vi "TEG P116x1_Write_Manual.vi"(8 "error in (no error)":errorcluster, 9 "NewRT":dbl, 10 "NewSP":dbl, 11 "Comunicaciones":T1={"EUROTHERM"="ASRL6::INSTR", "eur"=FALSE, "ESP32"="ASRL6::INSTR", "esp"=FALSE}) -> (0 "error out":errorcluster, 1 "NewRT 2":dbl, 2 "NewSP 2":dbl)   [LabVIEW 2017]
uses:
  cTEG COMMS.ctl
  Eurotherm_New_Module.ctl
  TEG TEST 2022 GLOBALES.vi
panel:
  out "PV":dbl
  out "WorKSP":dbl
  out "TargetSP":dbl
  in  "Cancel":bool
  in  "Write":bool
  out "Enable(T)":bool=TRUE
  out "VISA Promux":refnum<visa-resource-name>
  # "Programando controlador P116"
  # "C"
  # "C/min"
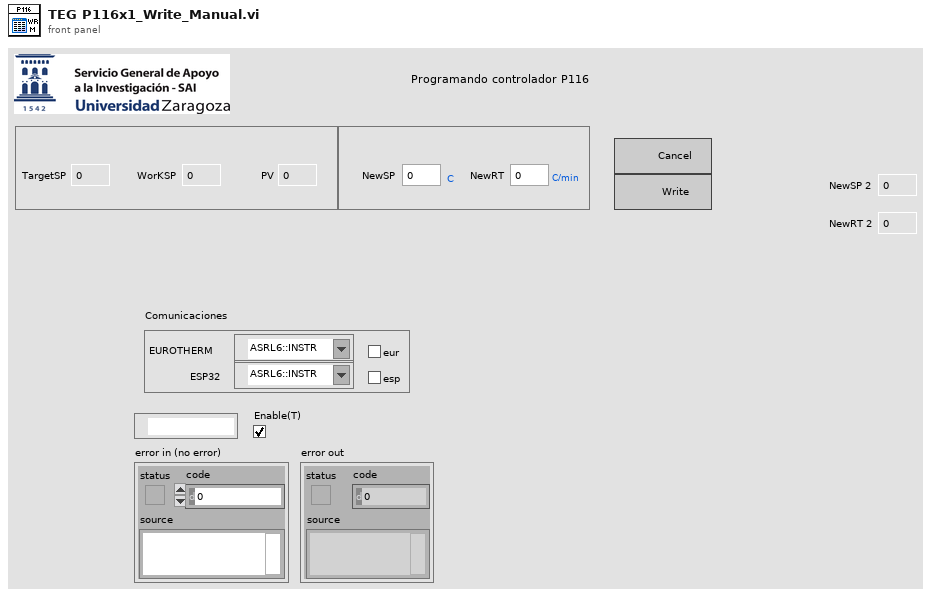
[diagram p1: front panel]
types:
  T1 = typedef "cTEG COMMS.ctl" = cluster{"EUROTHERM":refnum<visa-resource-name>, "eur":bool, "ESP32":refnum<visa-resource-name>, "esp":bool}
  T2 = typedef "TEG P116x1.ctl" = cluster{"TargetSP":dbl, "WorkingSP":dbl, "Temperatura":dbl, "RateSP":dbl, "Potencia":dbl}
  T3 = typedef "Eurotherm_New_Module.ctl" = enum16{"Initialize", "Write SP", "Read SP+PV", "Write Rate", "Set P", "Set I", "Set D", "Shutdown"}
  T4 = enum16{"Add 1", "Add 2", "Add 10", "Add 11", "Add 12", "Add 13"}
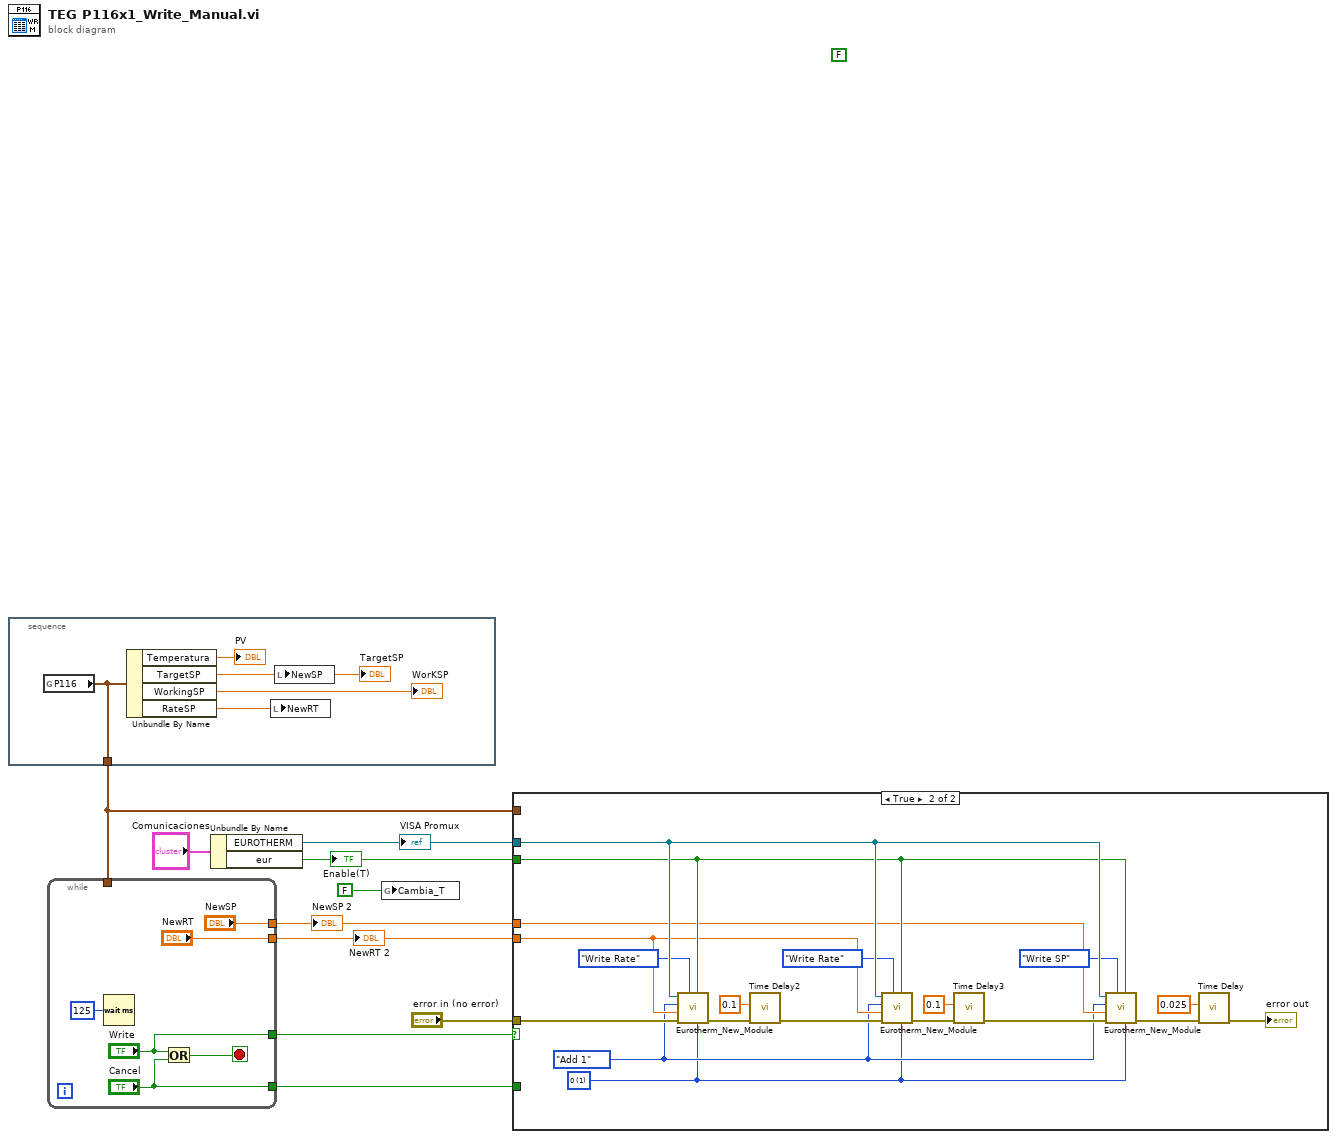
[diagram p0: block diagram]
diagram:
  (unwired) FALSE
  n1 = stacked-sequence {
    tunnel: [w12] -> w4
    frame #0 {
      n2 = global read "TEG TEST 2022 GLOBALES.vi" "P116"() -> (w12:T2)
      n3 = Unbundle By Name(w12) -> ("Temperatura"=→"PV":dbl, "TargetSP"=w13:dbl, "WorkingSP"=→"WorKSP":dbl, "RateSP"=w11:dbl)
      "TargetSP" <- w13
      n4 = local write "NewRT"(w11) -> ()
      n5 = local write "NewSP"(w13) -> ()
    }
  }
  n6 = while {
    tunnel: ["Cancel"] -> w9
    tunnel: ["NewSP"] -> w1
    tunnel: ["NewRT"] -> w2
    tunnel: ["Write"] -> w7
    tunnel: w4 -> [_]
    stop <- w16 stop-if-true
    n7 = Wait (ms)(milliseconds to wait=u32 125) -> ()  [unwired: 1 out]
    n8 = Or(x="Write", y="Cancel") -> (x .or. y?=w16:bool)
  }
  "NewSP 2" <- w1
  "NewRT 2" <- w2
  n9 = Unbundle By Name("Comunicaciones") -> ("EUROTHERM"=w5:refnum<visa-resource-name>, "eur"=w10:bool)
  "Enable(T)" <- w10
  "VISA Promux" <- w5
  n10 = global write "TEG TEST 2022 GLOBALES.vi" "Cambia_T"(FALSE ("ChangeT")) -> ()
  n11 = case shown="True" w7 {
    tunnel: w10 -> [_ w39]
    tunnel: w9 -> [_ _]
    tunnel: "error in (no error)" -> [_ w37]
    tunnel: w1 -> [_ w35]
    tunnel: w2 -> [_ w36]
    tunnel: w5 -> [_ w40]
    tunnel: w4 -> [_ _]
    frame False {
    }
    frame True {
      w23 = T4."Add 1" ("Address")
      w22 = u16 1 items=["0"=1, "1"=10, "2"=100] ("Decimales")
      n12 = call "Eurotherm_New_Module.vi"("Decimales"=w22, "Eurotherm (T:Enable)"=w39, "Command"=Eurotherm_New_Module."Write Rate", "error in (no error)"=w37, "Value"=w36, "Address"=w23, "VISA resource name"=w40) -> ("error out"=w30:errorcluster)  [unwired: 3 in, 1 out]
      n13 = call "Time Delay2"("error in (no error)"=w30, "Delay Time (s)"=0.1) -> ("error out"=w25:errorcluster)  [unwired: 9 in]
      n14 = call "Eurotherm_New_Module.vi"("Decimales"=w22, "Eurotherm (T:Enable)"=w39, "Command"=Eurotherm_New_Module."Write Rate", "error in (no error)"=w25, "Value"=w36, "Address"=w23, "VISA resource name"=w40) -> ("error out"=w27:errorcluster)  [unwired: 3 in, 1 out]
      n15 = call "Time Delay3"("error in (no error)"=w27, "Delay Time (s)"=0.1) -> ("error out"=w24:errorcluster)  [unwired: 9 in]
      n16 = call "Eurotherm_New_Module.vi"("Decimales"=w22, "Eurotherm (T:Enable)"=w39, "Command"=Eurotherm_New_Module."Write SP", "error in (no error)"=w24, "Value"=w35, "Address"=w23, "VISA resource name"=w40) -> ("error out"=w31:errorcluster)  [unwired: 3 in, 1 out]
      n17 = call "Time Delay"("error in (no error)"=w31, "Delay Time (s)"=0.025) -> ("error out"=→"error out":errorcluster)  [unwired: 9 in]
    }
  }
